vi "0x2 RIO-OCU update receive.vi"() -> (2 "Local Network \nLoop Iterations":i64, 3 "Remote Network \nLoop Iterations":i64)   [LabVIEW 2011]
doc: "Runs in the OCU and recieves data sent by 0x2 RIO-OCU update recieve.vi for monitoring and debugging purposes."
uses:
  0x2 Typedefs/RIO-OCU update controls.ctl
  2-Think/2 Typedefs/generalized sensor status.ctl
  2-Think/2 Typedefs/indicator LED.ctl
  2-Think/2 Typedefs/generalized actuator status.ctl
  2-Think/2 Typedefs/Which Boat.ctl
  2-Think/2 Typedefs/robot velocity.ctl
  2-Think/2 Typedefs/UTM Location.ctl
  2-Think/2 Typedefs/heading.ctl
  2-Think/2 Typedefs/rate of turn.ctl
  2-Think/2 Typedefs/pitch and roll.ctl
  2-Think/2 Typedefs/apparent wind.ctl
  2-Think/2 Typedefs/apparent wind speed.ctl
  2-Think/2 Typedefs/apparent wind direction.ctl
  2-Think/2 Typedefs/Velocity.ctl
  2-Think/2 Typedefs/absolute wind direction.ctl
  2-Think/2 Typedefs/absolute wind speed.ctl
  2-Think/2 Typedefs/absolute water current vector.ctl
  2-Think/2 Typedefs/rudder angle.ctl
  2-Think/2 Typedefs/sail setpt.ctl
  0x2 Typedefs/manual override.ctl
  2-Think/2 Typedefs/setpoints to boat.ctl
  0x2 Typedefs/Waypoints List.ctl
  0x2 Typedefs/ocuWaypoint.ctl
  0x2 Typedefs/waypointTypes.ctl
  0x2 Typedefs/Current Waypoint.ctl
  2-Think/2 Globals/2 Global.vi
panel:
  in  "Monitored Items from RIO":T1 {"Robot Pitch/Roll"."Roll" format="%05.1f"; "Robot Pitch/Roll"."Pitch" format="%05.1f"; "Robot\nRate of Turn" format="%05.1f"; "Robot\nHeading" format="%05.1f"}
  # "How Am I?"
  # "Where Am I?"
  # "Path Planning"
  # "From Planning Functions"
  # "(this is not a cluster because subitems\nare generated in parallel code)"
  # "What's Around Me?"
  # "As Measured"
  # "As Measured"
  # "Loop Rates"
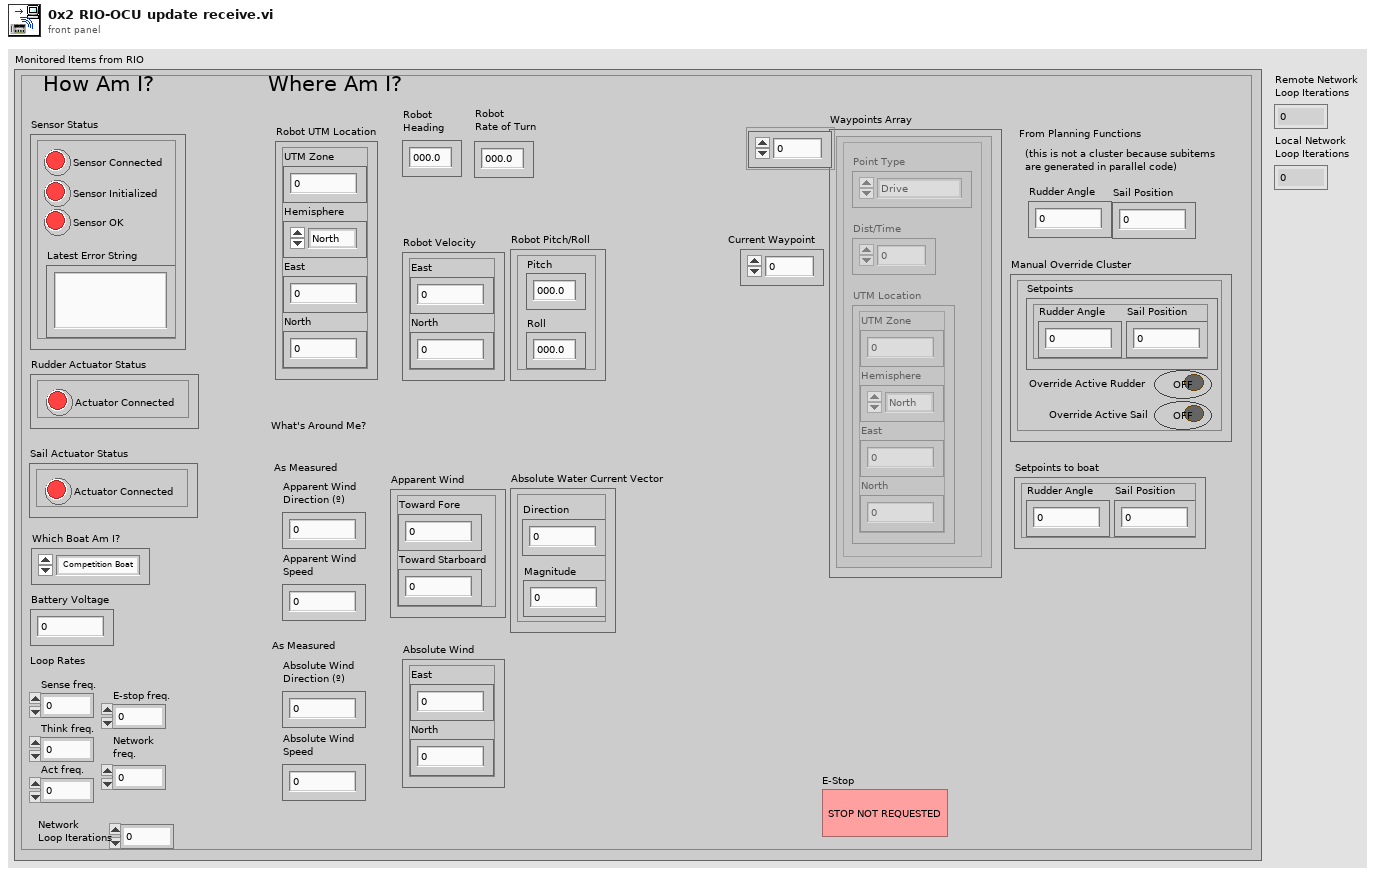
[diagram p1: front panel]
types:
  T1 = typedef "RIO-OCU update controls.ctl" = cluster{"Sensor Status":T2, "Battery Voltage":dbl, "Rudder Actuator Status":T4, "Sail Actuator Status":T4, "Which Boat Am I?":T5, "Robot Velocity":T6, "Robot UTM Location":T7, "Robot\nHeading ":T8, "Robot\nRate of Turn":T9, "Robot Pitch/Roll":T10, "Apparent Wind":T11, "Apparent Wind\nSpeed":T12, "Apparent Wind\nDirection (º)":T13, "Absolute Wind":T14, "Absolute Wind\nDirection (º)":T15, "Absolute Wind\nSpeed":T16, "Absolute Water Current Vector":T17, "Rudder Angle":T18, "Sail Position":T19, "Manual Override Cluster":T20, "Setpoints to boat":T21, "Waypoints Array":T22, "Current Waypoint":T25, "Think freq.":dbl, "Sense freq.":dbl, "Act freq.":dbl, "E-stop freq.":dbl, "Network \nfreq.":dbl, "Network \nLoop Iterations":i64, "E-Stop":bool}
  T2 = typedef "generalized sensor status.ctl" = cluster{"Sensor Connected":T3, "Sensor Initialized":T3, "Sensor OK":T3, "Latest Error String":string}
  T3 = typedef "indicator LED.ctl" = bool
  T4 = typedef "generalized actuator status.ctl" = cluster{"Actuator Connected":T3}
  T5 = typedef "Which Boat.ctl" = enum16{"Competition Boat", "Small RC", "Simulation"}
  T6 = typedef "robot velocity.ctl" = cluster{"East":dbl, "North":dbl}
  T7 = typedef "UTM Location.ctl" = cluster{"UTM Zone":dbl, "Hemisphere":enum16{"North", "South"}, "East":dbl, "North":dbl}
  T8 = typedef "heading.ctl" = dbl
  T9 = typedef "rate of turn.ctl" = dbl
  T10 = typedef "pitch and roll.ctl" = cluster{"Pitch":dbl, "Roll":dbl}
  T11 = typedef "apparent wind.ctl" = cluster{"Toward Fore":dbl, "Toward Starboard":dbl}
  T12 = typedef "apparent wind speed.ctl" = dbl
  T13 = typedef "apparent wind direction.ctl" = dbl
  T14 = typedef "Velocity.ctl" = cluster{"East":dbl, "North":dbl}
  T15 = typedef "absolute wind direction.ctl" = dbl
  T16 = typedef "absolute wind speed.ctl" = dbl
  T17 = typedef "absolute water current vector.ctl" = cluster{"Direction":T13, "Magnitude":T13}
  T18 = typedef "rudder angle.ctl" = dbl
  T19 = typedef "sail setpt.ctl" = dbl
  T20 = typedef "manual override.ctl" = cluster{"Override Active Rudder":bool, "Setpoints":T21, "Override Active Sail":bool}
  T21 = typedef "setpoints to boat.ctl" = cluster{"Sail Position":T19, "Rudder Angle":T18}
  T22 = typedef "Waypoints List.ctl" = T23[]
  T23 = typedef "ocuWaypoint.ctl" = cluster{"Point Type":T24, "Dist/Time":dbl, "UTM Location":T7}
  T24 = typedef "waypointTypes.ctl" = enum16{"Drive", "Round Port", "Round Starboard", "Stay"}
  T25 = typedef "Current Waypoint.ctl" = i32
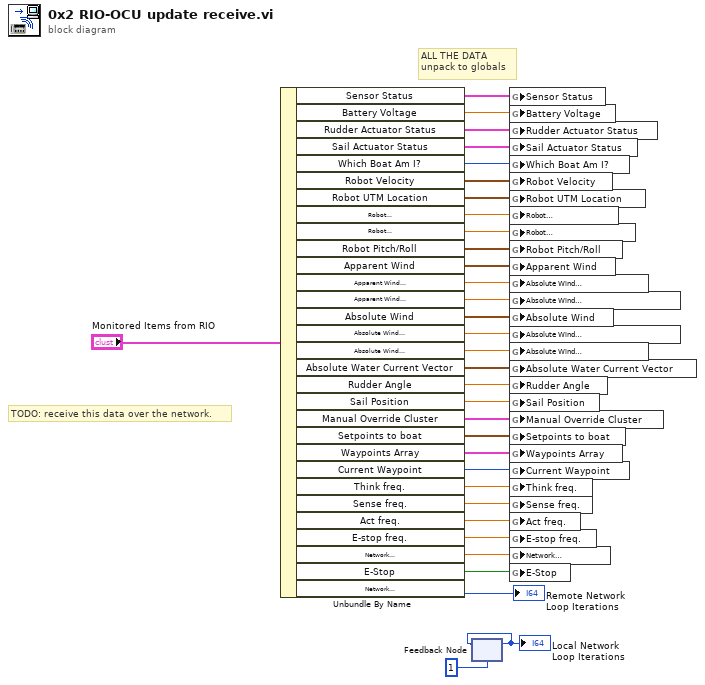
[diagram p0: block diagram]
diagram:
  # "ALL THE DATA\nunpack to globals"
  # "TODO: receive this data over the network."
  n1 = Unbundle By Name("Monitored Items from RIO") -> ("Sensor Status"=w12:T2, "Battery Voltage"=w25:dbl, "Rudder Actuator Status"=w11:T4, "Sail Actuator Status"=w10:T4, "Which Boat Am I?"=w13:T5, "Robot Velocity"=w9:T6, "Robot UTM Location"=w8:T7, "Robot\nHeading"=w14:T8, "Robot\nRate of Turn"=w15:T9, "Robot Pitch/Roll"=w7:T10, "Apparent Wind"=w6:T11, "Apparent Wind\nSpeed"=w19:T12, "Apparent Wind\nDirection (º)"=w18:T13, "Absolute Wind"=w5:T14, "Absolute Wind\nDirection (º)"=w17:T15, "Absolute Wind\nSpeed"=w16:T16, "Absolute Water Current Vector"=w4:T17, "Rudder Angle"=w20:T18, "Sail Position"=w26:T19, "Manual Override Cluster"=w24:T20, "Setpoints to boat"=w21:T21, "Waypoints Array"=w22:T22, "Current Waypoint"=w23:T25, "Think freq."=w32:dbl, "Sense freq."=w31:dbl, "Act freq."=w30:dbl, "E-stop freq."=w29:dbl, "Network \nfreq."=w28:dbl, "E-Stop"=w27:bool, "Network \nLoop Iterations"=→"Remote Network \nLoop Iterations":i64)
  n2 = feedback #1(i64 1 ("Local Network \nLoop Iterations 2")) -> (w2:i64)
  "Local Network \nLoop Iterations" <- w2
  n3 = feedback-in #1(w2) -> ()
  n4 = global write "2 Global.vi" "Sensor Status"(w12) -> ()
  n5 = global write "2 Global.vi" "Battery Voltage"(w25) -> ()
  n6 = global write "2 Global.vi" "Rudder Actuator Status"(w11) -> ()
  n7 = global write "2 Global.vi" "Sail Actuator Status"(w10) -> ()
  n8 = global write "2 Global.vi" "Which Boat Am I?"(w13) -> ()
  n9 = global write "2 Global.vi" "Robot Velocity"(w9) -> ()
  n10 = global write "2 Global.vi" "Robot UTM Location"(w8) -> ()
  n11 = global write "2 Global.vi" "Robot\nHeading"(w14) -> ()
  n12 = global write "2 Global.vi" "Robot\nRate of Turn"(w15) -> ()
  n13 = global write "2 Global.vi" "Robot Pitch/Roll"(w7) -> ()
  n14 = global write "2 Global.vi" "Apparent Wind"(w6) -> ()
  n15 = global write "2 Global.vi" "Absolute Wind\nSpeed"(w19) -> ()
  n16 = global write "2 Global.vi" "Absolute Wind\nDirection (º)"(w18) -> ()
  n17 = global write "2 Global.vi" "Absolute Wind"(w5) -> ()
  n18 = global write "2 Global.vi" "Absolute Wind\nDirection (º)"(w17) -> ()
  n19 = global write "2 Global.vi" "Absolute Wind\nSpeed"(w16) -> ()
  n20 = global write "2 Global.vi" "Absolute Water Current Vector"(w4) -> ()
  n21 = global write "2 Global.vi" "Rudder Angle"(w20) -> ()
  n22 = global write "2 Global.vi" "Sail Position"(w26) -> ()
  n23 = global write "2 Global.vi" "Manual Override Cluster"(w24) -> ()
  n24 = global write "2 Global.vi" "Setpoints to boat"(w21) -> ()
  n25 = global write "2 Global.vi" "Waypoints Array"(w22) -> ()
  n26 = global write "2 Global.vi" "Current Waypoint"(w23) -> ()
  n27 = global write "2 Global.vi" "Think freq."(w32) -> ()
  n28 = global write "2 Global.vi" "Sense freq."(w31) -> ()
  n29 = global write "2 Global.vi" "Act freq."(w30) -> ()
  n30 = global write "2 Global.vi" "E-stop freq."(w29) -> ()
  n31 = global write "2 Global.vi" "Network \nfreq."(w28) -> ()
  n32 = global write "2 Global.vi" "E-Stop"(w27) -> ()
